vi "In Relative Range and Coerce.vi"(7 "relative base":dbl, 9 "relative lower limit":dbl, 10 "x":dbl, 11 "relative upper limit":dbl) -> (2 "coerced(x)":dbl, 3 "In Range?":bool)   [LabVIEW 2020, in "varilib.lvlib"]
doc: "Determines whether x falls within a range specified by the base, relative upper limit and relative lower limit inputs and optionally coerces the value to fall within the range. Limits are relative, i.e. vi tests if x is in range of base*(1+upper relative limit) and base*(1-lower relative limit). Adds machine precision to prevent round-off error of floating numbers. Limits are expected to be positive."
uses:
  varilib.lvlib
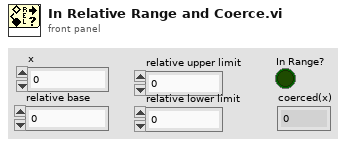
[diagram p1: front panel]
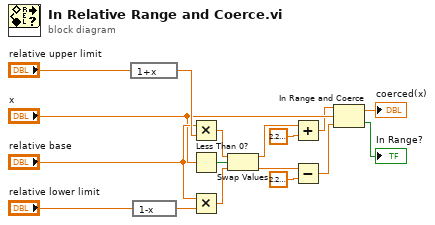
[diagram p0: block diagram]
diagram:
  n1 = expression code="1+x"("relative upper limit") -> (w16:dbl)
  n2 = expression code="1-x"("relative lower limit") -> (w17:dbl)
  n3 = Multiply(x="relative base", y=w16) -> (x*y=w8:dbl)
  n4 = Less Than 0?(x="x") -> (x < 0?=w4:bool)
  n5 = Multiply(x="relative base", y=w17) -> (x*y=w6:dbl)
  n6 = Swap Values(12:w8, 13:w4, 14:w6) -> (1:w7:dbl, 3:w5:dbl)
  n7 = Add(x=w7, y=2.220446049250313e-16) -> (x+y=w3:dbl)
  n8 = Subtract(x=w5, y=2.220446049250313e-16) -> (x-y=w2:dbl)
  n9 = In Range and Coerce(upper limit=w3, x="x", lower limit=w2) -> (coerced(x)=→"coerced(x)":dbl, In Range?=→"In Range?":bool)
